vi "Contex Menu Selection.vi"(8 "error in (no error)":errorcluster, 10 "MenuItem":string, 11 "HIJ IMAQdx Display in":refnum<class "HIJ IMAQdx Display.lvclass">) -> (0 "error out":errorcluster, 3 "HIJ IMAQdx Display out":refnum<class "HIJ IMAQdx Display.lvclass">)   [LabVIEW 2014, in "HIJ IMAQdx Display.lvlib" / "HIJ IMAQdx Display.lvclass"]
uses:
  HIJ IMAQdx Display.lvclass
  HIJ Vision Display/HIJ Vision Display/HIJ Vision Display.lvclass
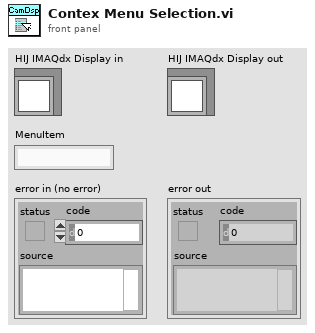
[diagram p1: front panel]
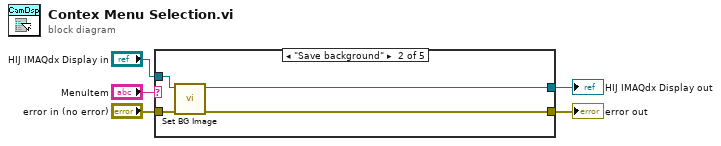
[diagram p0: block diagram]
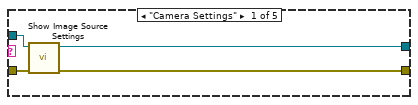
[diagram p2: hidden frame]
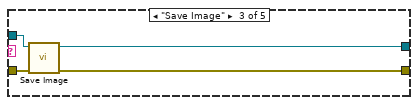
[diagram p3: hidden frame]
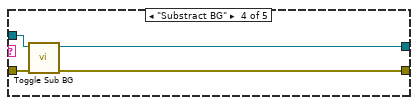
[diagram p4: hidden frame]
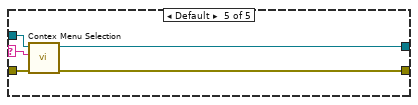
[diagram p5: hidden frame]
diagram:
  n1 = case shown="\"Save background\"" "MenuItem" {
    selector: "MenuItem" -> [_ _ _ _ w23]
    tunnel: "HIJ IMAQdx Display in" -> [w9 w13 w17 w21 w26]
    tunnel: "error in (no error)" -> [w8 w11 w14 w18 w25]
    tunnel: [w6 w12 w16 w20 w24] -> w3
    tunnel: [w7 w10 w15 w19 w22] -> w1
    frame "Camera Settings" {
      n2 = call-dynamic "Show Image Source Settings.vi"("error in (no error)"=w8, "AF IMAQ Display in"=w9) -> ("error out"=w7:errorcluster, "AF IMAQ Display out"=w6:refnum<class "HIJ IMAQdx Display.lvclass">)  [unwired: 8 in]
    }
    frame "Save background" {
      n3 = call "Set BG Image.vi"("error in (no error)"=w11, "IMAQ Display in"=w13) -> ("error out"=w10:errorcluster, "IMAQ Display out"=w12:refnum<class "HIJ IMAQdx Display.lvclass">)  [unwired: 8 in]
    }
    frame "Save Image" {
      n4 = call-dynamic "Save Image.vi"("error in (no error)"=w14, "IMAQ Display in"=w17) -> ("error out"=w15:errorcluster, "IMAQ Display out"=w16:refnum<class "HIJ IMAQdx Display.lvclass">)  [unwired: 8 in]
    }
    frame "Substract BG" {
      n5 = call "Toggle Sub BG.vi"("error in (no error)"=w18, "IMAQ Display in"=w21) -> ("error out"=w19:errorcluster, "IMAQ Display out"=w20:refnum<class "HIJ IMAQdx Display.lvclass">)  [unwired: 8 in]
    }
    frame Default {
      n6 = call-parent "Contex Menu Selection.vi"("error in (no error)"=w25, "MenuItem"=w23, "HIJ Vision Display in"=w26) -> ("error out"=w22:errorcluster, "HIJ Vision Display out"=w24:refnum<class "HIJ IMAQdx Display.lvclass">)  [unwired: 7 in]
    }
  }
  "error out" <- w1
  "HIJ IMAQdx Display out" <- w3
